vi "Set Base Path.vi"(8 "error in (no error)":errorcluster, 9 "Encode?":bool, 10 "base-path":string, 11 "URI in":refnum<class "URI.lvclass">) -> (0 "error out":errorcluster, 3 "URI out":refnum<class "URI.lvclass">)   [LabVIEW 2013, in "openURI.lvlib" / "URI.lvclass"]
uses:
  URI.lvclass
  URI.lvclass/URI.ctl
  utilities/isHEXDigit.vi
  components/path/URI-Component.Path.lvclass
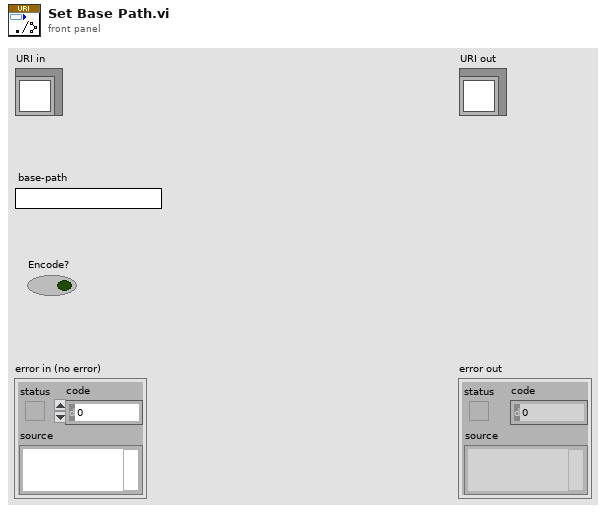
[diagram p1: front panel]
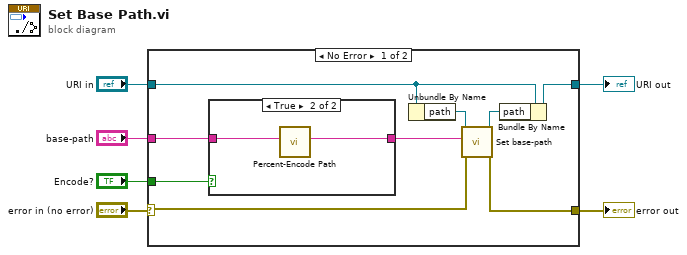
[diagram p0: block diagram]
diagram:
  n1 = case shown="No Error" "error in (no error)" {
    selector: "error in (no error)" -> [w8 w20]
    tunnel: [w7 w20] -> w5
    tunnel: [w12 w19] -> w3
    tunnel: "URI in" -> [w13 w19]
    tunnel: "base-path" -> [w14 _]
    tunnel: "Encode?" -> [w15 _]
    frame No Error {
      n2 = case shown="True" w15 {
        tunnel: [w16 w17] -> w11
        tunnel: w14 -> [w16 w18]
        frame False {
        }
        frame True {
          n3 = call "Percent-Encode Path.vi"("Path"=w18) -> ("Pct-Encoded Path"=w17:string)  [unwired: 10 in]
        }
      }
      n4 = Unbundle By Name(w13) -> ("path"=w10:refnum<class "URI-Component.Path.lvclass">)
      n5 = call "Set base-path.vi"("error in (no error)"=w8, "base-path"=w11, "URI-Component.Path in"=w10) -> ("error out"=w7:errorcluster, "URI-Component.Path out"=w9:refnum<class "URI-Component.Path.lvclass">)  [unwired: 7 in]
      n6 = Bundle By Name(cluster=w13, "path"=w9) -> (w12:refnum<class "URI.lvclass">)
    }
    frame Error {
    }
  }
  "error out" <- w5
  "URI out" <- w3
